vi "tm3samp_10_dualsync.vi"() -> ()   [LabVIEW 2011]
panel:
  out "Camera Model":string
  out "Image":u16[][](graph)
  in  "capture":bool
  in  "Quit":bool
  out "Error Out":errorcluster {"code" format="%.0x"}
  # "This is an example of one way\nto synchronize two of the same\nmodel cameras."
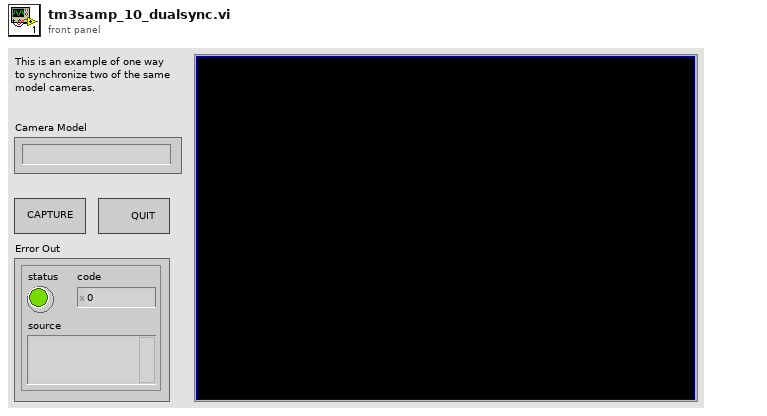
[diagram p1: front panel]
types:
  T1 = cluster{"height":u32, "width":u32, "datatype":u32}
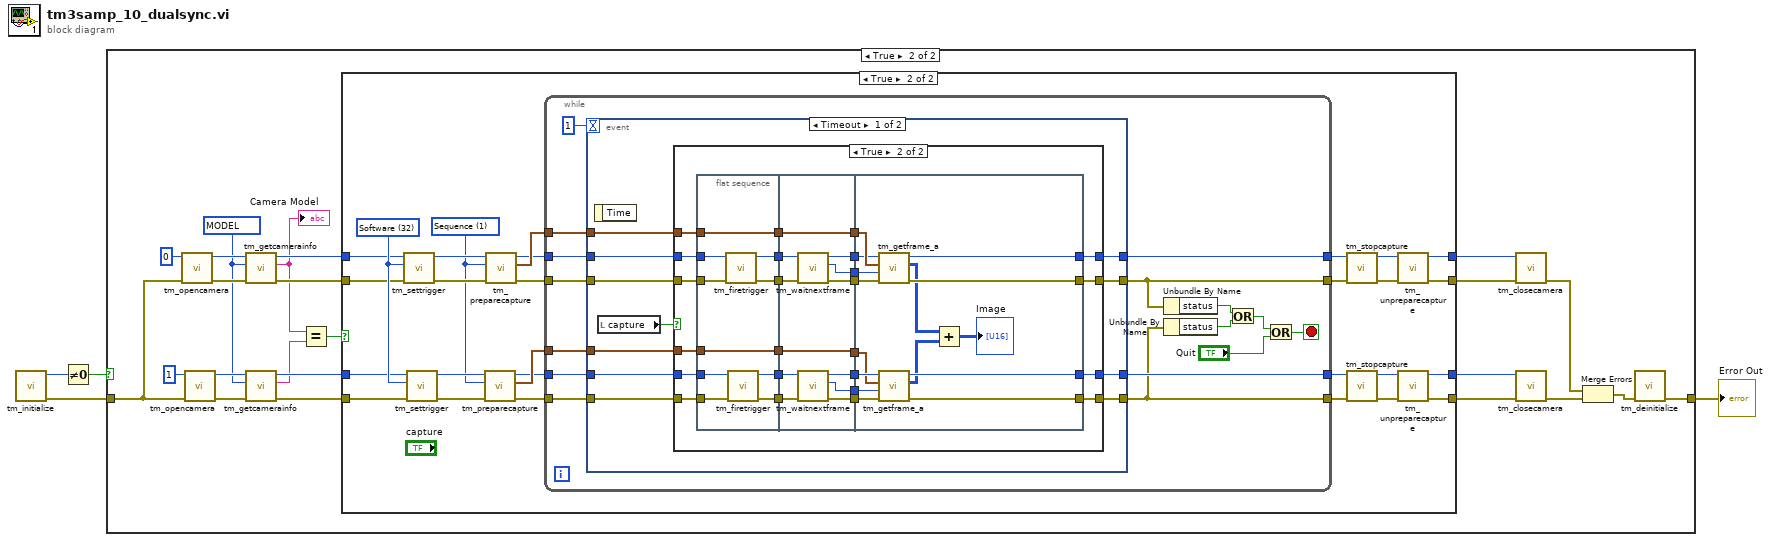
[diagram p0: block diagram]
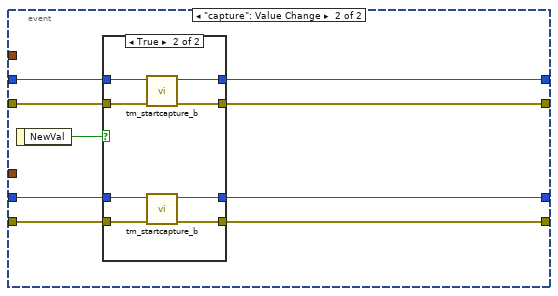
[diagram p5: hidden frame]
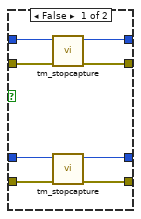
[diagram p6: hidden frame]
diagram:
  n1 = call <userlib>:"tm_initialize.vi"() -> ("error out"=w1:errorcluster, "Number Of Cameras"=w2:u32)  [unwired: 8 in, 2 out]
  n2 = Not Equal To 0?(x=w2) -> (x != 0?=w4:bool)
  n3 = case shown="True" w4 {
    tunnel: w1 -> [w5 w25]
    tunnel: [w5 w27] -> w3
    frame False {
    }
    frame True {
      w17 = u32 67109124 items=["BUS"=67109121, "CAMERA ID"=67109122, "VENDOR"=67109123, "MODEL"=67109124, "CAMERA VERSION"=67109125, "DRIVER VERSION"=67109126, "MODULE VERSIOIN"=67109127, "DCAMAPI VERSION"=67109128] ("Info ID")
      n4 = call <userlib>:"tm_opencamera.vi"("error in (no error)"=w25, "Camera Index"=u32 0) -> ("error out"=w20:errorcluster, "Handle out"=w21:u32)  [unwired: 7 in, 1 out]
      n5 = call <userlib>:"tm_opencamera.vi"("error in (no error)"=w25, "Camera Index"=u32 1) -> ("error out"=w18:errorcluster, "Handle out"=w19:u32)  [unwired: 7 in, 1 out]
      n6 = call <userlib>:"tm_getcamerainfo.vi"("error in (no error)"=w20, "Info ID"=w17, "Handle in"=w21) -> ("error out"=w14:errorcluster, "String"=w8:string, "Handle out"=w13:u32)  [unwired: 6 in]
      "Camera Model" <- w8
      n7 = call <userlib>:"tm_getcamerainfo.vi"("error in (no error)"=w18, "Info ID"=w17, "Handle in"=w19) -> ("error out"=w15:errorcluster, "String"=w7:string, "Handle out"=w16:u32)  [unwired: 6 in]
      n8 = Equal?(x=w8, y=w7) -> (x = y?=w6:bool)
      n9 = case shown="True" w6 {
        tunnel: w16 -> [w32 w42]
        tunnel: w15 -> [w31 w41]
        tunnel: w14 -> [w30 w37]
        tunnel: w13 -> [w29 w38]
        tunnel: [w32 w44] -> w12
        tunnel: [w31 w43] -> w11
        tunnel: [w30 w39] -> w10
        tunnel: [w29 w40] -> w9
        frame False {
        }
        frame True {
          w45 = u32 32 items=["Internal"=1, "External Edge"=2, "External Level"=4, "Software"=32, "Fast Repetition"=64, "TDI"=128, "Trigger Start"=512, "Sync Readout"=1024] ("Trigger Mode")
          w46 = 1 items=["Snap", "Sequence"] ("Capture mode")
          n10 = call <userlib>:"tm_settrigger.vi"("error in (no error)"=w37, "Trigger Mode"=w45, "Handle in"=w38) -> ("error out"=w52:errorcluster, "Handle out"=w53:u32)  [unwired: 7 in]
          n11 = call <userlib>:"tm_settrigger.vi"("error in (no error)"=w41, "Trigger Mode"=w45, "Handle in"=w42) -> ("error out"=w54:errorcluster, "Handle out"=w55:u32)  [unwired: 7 in]
          n12 = call <userlib>:"tm_preparecapture.vi"("error in (no error)"=w54, "Capture mode"=w46, "Handle in"=w55) -> ("error out"=w33:errorcluster, "Buffer Info"=w60:T1, "Handle out"=w34:u32)  [unwired: 5 in, 1 out]
          n13 = call <userlib>:"tm_preparecapture.vi"("error in (no error)"=w52, "Capture mode"=w46, "Handle in"=w53) -> ("error out"=w36:errorcluster, "Buffer Info"=w51:T1, "Handle out"=w35:u32)  [unwired: 5 in, 1 out]
          n14 = while {
            tunnel: [w74] -> w59
            tunnel: [w66] -> w58
            tunnel: w34 -> [w76]
            tunnel: w33 -> [w75]
            tunnel: w60 -> [w73]
            tunnel: w35 -> [w70]
            tunnel: w36 -> [w69]
            tunnel: w51 -> [w68]
            tunnel: [w65] -> w47
            tunnel: [w67] -> w48
            stop <- w63 stop-if-true
            n15 = event shown="[0] Timeout" {
              selector: _ -> [_ _]
              dyn-events: _ -> [_ _]
              timeout: 1 -> [_ _]
              tunnel: w76 -> [w82 w160]
              tunnel: w75 -> [w81 w159]
              tunnel: [w78 w158] -> w74
              tunnel: [w77 w157] -> w66
              tunnel: w73 -> [w83 _]
              tunnel: w70 -> [w85 w156]
              tunnel: w68 -> [w86 _]
              tunnel: w69 -> [w84 w155]
              tunnel: [w79 w153] -> w67
              tunnel: [w80 w154] -> w65
              event Timeout {
                n16 = event-data() -> ()  [unwired: 1 in, 1 out]
                n17 = local read "capture"() -> (w87:bool)
                n18 = case shown="True" w87 {
                  tunnel: w86 -> [_ w103]
                  tunnel: w85 -> [w91 w102]
                  tunnel: w84 -> [w90 w101]
                  tunnel: w83 -> [_ w100]
                  tunnel: w82 -> [w88 w99]
                  tunnel: w81 -> [w89 w98]
                  tunnel: [w90 w97] -> w80
                  tunnel: [w91 w96] -> w79
                  tunnel: [w88 w95] -> w78
                  tunnel: [w89 w94] -> w77
                  frame False {
                  }
                  frame True {
                    n19 = flat-sequence {
                      tunnel: w99 -> [w125]
                      tunnel: w98 -> [w124]
                      tunnel: [w123] -> w115
                      tunnel: [w122] -> w114
                      tunnel: w100 -> [w121]
                      tunnel: [w121] -> w113
                      tunnel: w103 -> [w120]
                      tunnel: [w120] -> w112
                      tunnel: w102 -> [w119]
                      tunnel: [w117] -> w111
                      tunnel: w101 -> [w118]
                      tunnel: [w116] -> w110
                      tunnel: w115 -> [w134]
                      tunnel: w114 -> [w135]
                      tunnel: w113 -> [w128]
                      tunnel: w112 -> [w133]
                      tunnel: w111 -> [w136]
                      tunnel: w110 -> [w137]
                      tunnel: [w133] -> w109
                      tunnel: [w132] -> w108
                      tunnel: [w131] -> w107
                      tunnel: [w130] -> w106
                      tunnel: [w129] -> w105
                      tunnel: [w128] -> w104
                      tunnel: [w126] -> w93
                      tunnel: [w127] -> w92
                      tunnel: w109 -> [w152]
                      tunnel: w108 -> [w150]
                      tunnel: w107 -> [w151]
                      tunnel: [w149] -> w96
                      tunnel: [w148] -> w97
                      tunnel: w106 -> [w147]
                      tunnel: w105 -> [w146]
                      tunnel: w104 -> [w145]
                      tunnel: [w144] -> w95
                      tunnel: [w143] -> w94
                      tunnel: w93 -> [w142]
                      tunnel: w92 -> [w141]
                      frame #0 {
                        n20 = call <userlib>:"tm_firetrigger.vi"("error in (no error)"=w118, "Handle in"=w119) -> ("error out"=w116:errorcluster, "Handle out"=w117:u32)  [unwired: 8 in]
                        n21 = call <userlib>:"tm_firetrigger.vi"("error in (no error)"=w124, "Handle in"=w125) -> ("error out"=w122:errorcluster, "Handle out"=w123:u32)  [unwired: 8 in]
                      }
                      frame #1 {
                        n22 = call <userlib>:"tm_waitnextframe.vi"("error in (no error)"=w137, "Handle in"=w136) -> ("error out"=w131:errorcluster, "Frame Index"=w126:i32, "Handle out"=w132:u32)  [unwired: 6 in, 1 out]
                        n23 = call <userlib>:"tm_waitnextframe.vi"("error in (no error)"=w135, "Handle in"=w134) -> ("error out"=w129:errorcluster, "Frame Index"=w127:i32, "Handle out"=w130:u32)  [unwired: 6 in, 1 out]
                      }
                      frame #2 {
                        n24 = call <userlib>:"tm_getframe_a.vi"("error in (no error)"=w151, "Frame Index"=w142, "Buffer Info"=w152, "Handle in"=w150) -> ("error out"=w148:errorcluster, "Data 16"=w140:u16[][], "Handle out"=w149:u32)  [unwired: 3 in, 2 out]
                        n25 = call <userlib>:"tm_getframe_a.vi"("error in (no error)"=w146, "Frame Index"=w141, "Buffer Info"=w145, "Handle in"=w147) -> ("error out"=w143:errorcluster, "Data 16"=w139:u16[][], "Handle out"=w144:u32)  [unwired: 3 in, 2 out]
                        n26 = Add(x=w140, y=w139) -> (x+y=→"Image":u16[][])
                      }
                    }
                  }
                }
              }
              event "capture": Value Change {
                n27 = event-data() -> ("NewVal"=w161:bool)  [unwired: 1 in]
                n28 = case shown="True" w161 {
                  tunnel: w160 -> [w169 w177]
                  tunnel: w159 -> [w168 w176]
                  tunnel: [w167 w175] -> w158
                  tunnel: [w166 w174] -> w157
                  tunnel: w156 -> [w164 w173]
                  tunnel: w155 -> [w165 w172]
                  tunnel: [w163 w171] -> w153
                  tunnel: [w162 w170] -> w154
                  frame False {
                    n29 = call <userlib>:"tm_stopcapture.vi"("error in (no error)"=w165, "Handle in"=w164) -> ("error out"=w162:errorcluster, "Handle out"=w163:u32)  [unwired: 8 in]
                    n30 = call <userlib>:"tm_stopcapture.vi"("error in (no error)"=w168, "Handle in"=w169) -> ("error out"=w166:errorcluster, "Handle out"=w167:u32)  [unwired: 8 in]
                  }
                  frame True {
                    n31 = call <userlib>:"tm_startcapture_b.vi"("error in (no error)"=w172, "Handle in"=w173) -> ("error out"=w170:errorcluster, "Handle out"=w171:u32)  [unwired: 8 in]
                    n32 = call <userlib>:"tm_startcapture_b.vi"("error in (no error)"=w176, "Handle in"=w177) -> ("error out"=w174:errorcluster, "Handle out"=w175:u32)  [unwired: 8 in]
                  }
                }
              }
            }
            n33 = Unbundle By Name(w65) -> ("status"=w72:bool)
            n34 = Unbundle By Name(w66) -> ("status"=w64:bool)
            n35 = Or(x=w72, y=w64) -> (x .or. y?=w62:bool)
            n36 = Or(x=w62, y="Quit") -> (x .or. y?=w63:bool)
          }
          n37 = call <userlib>:"tm_stopcapture.vi"("error in (no error)"=w47, "Handle in"=w48) -> ("error out"=w49:errorcluster, "Handle out"=w50:u32)  [unwired: 8 in]
          n38 = call <userlib>:"tm_stopcapture.vi"("error in (no error)"=w58, "Handle in"=w59) -> ("error out"=w56:errorcluster, "Handle out"=w57:u32)  [unwired: 8 in]
          n39 = call <userlib>:"tm_unpreparecapture.vi"("error in (no error)"=w49, "Handle in"=w50) -> ("error out"=w39:errorcluster, "Handle out"=w40:u32)  [unwired: 8 in]
          n40 = call <userlib>:"tm_unpreparecapture.vi"("error in (no error)"=w56, "Handle in"=w57) -> ("error out"=w43:errorcluster, "Handle out"=w44:u32)  [unwired: 8 in]
        }
      }
      n41 = call <userlib>:"tm_closecamera.vi"("error in (no error)"=w10, "Handle in"=w9) -> ("error out"=w24:errorcluster)  [unwired: 9 in]
      n42 = call <userlib>:"tm_closecamera.vi"("error in (no error)"=w11, "Handle in"=w12) -> ("error out"=w23:errorcluster)  [unwired: 9 in]
      n43 = Merge Errors(w24, w23) -> (w22:errorcluster)
      n44 = call <userlib>:"tm_deinitialize.vi"("error in (no error)"=w22) -> ("error out"=w27:errorcluster)  [unwired: 10 in]
    }
  }
  "Error Out" <- w3
